vi "Configure RF Output.vi"(4 "Enable Reverse Power Protection (T:Enable)":bool=TRUE, 6 "Enable Blanking (T:Enable)":bool=TRUE, 7 "Enable Modulation (T:Enable)":bool=TRUE, 8 "error in (no error)":errorcluster, 9 "Auto Blanking (T:Enable)":bool=TRUE, 10 "Enable RF Output (F:Disable)":bool, 11 "VISA resource name":refnum<visa-resource-name>) -> (0 "error out":errorcluster, 3 "VISA resource name out":refnum<visa-resource-name>)   [LabVIEW 2014, in "Agilent PSG MXG Series.lvlib"]
doc: "Configures RF output, modulation state, blanking, and RPP circuit of the signal generator."
uses:
  Agilent PSG MXG Series.lvlib
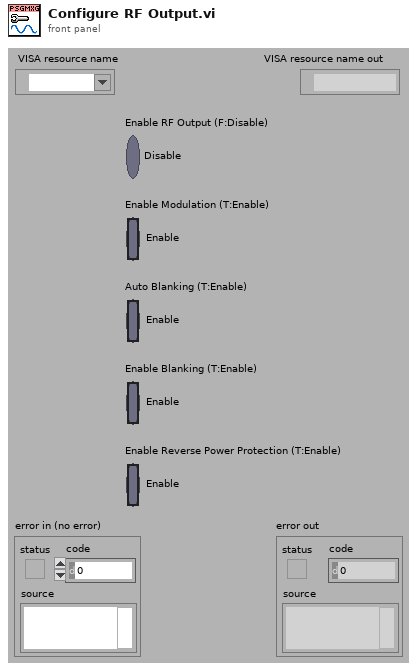
[diagram p1: front panel]
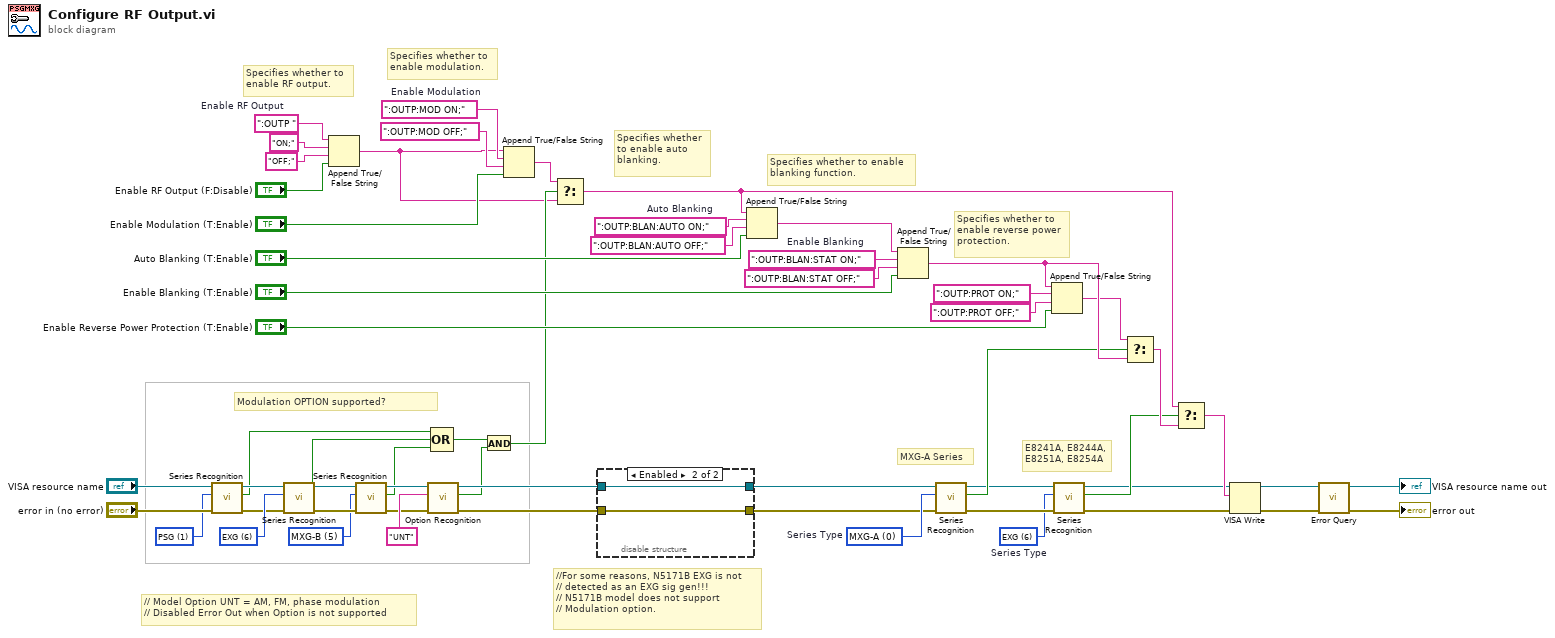
[diagram p0: block diagram]
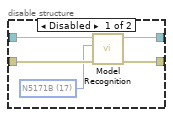
[diagram p2: hidden frame]
diagram:
  w2 = u16 1 items=["MXG-A", "PSG", "PSG-A", "PSG-C", "PSG-D", "MXG-B", "EXG"] ("Series Type (0: MXG)")
  w12 = u16 5 items=["MXG-A", "PSG", "PSG-A", "PSG-C", "PSG-D", "MXG-B", "EXG"] ("Series Type (0: MXG)")
  w23 = u16 6 items=["MXG-A", "PSG", "PSG-A", "PSG-C", "PSG-D", "MXG-B", "EXG"] ("Series Type")
  w24 = u16 6 items=["MXG-A", "PSG", "PSG-A", "PSG-C", "PSG-D", "MXG-B", "EXG"]  # Series Type
  w25 = u16 0 items=["MXG-A", "PSG", "PSG-A", "PSG-C", "PSG-D", "MXG-B", "EXG"]  # Series Type
  w36 = ":OUTP:BLAN:STAT ON;"  # Enable Blanking
  w51 = ":OUTP:BLAN:AUTO ON;"  # Auto Blanking
  w54 = ":OUTP:MOD ON;"  # Enable Modulation
  w58 = ":OUTP "  # Enable RF Output
  # "Modulation OPTION supported?"
  # "//For some reasons, N5171B EXG is not\n// detected as an EXG sig gen!!!\n// N5171B model does not support\n// Modulation option."
  # "// Model Option UNT = AM, FM, phase modulation\n// Disabled Error Out when Option is not supported"
  # "MXG-A Series"
  # "Specifies whether to\nenable reverse power\nprotection."
  # "Specifies whether to enable\nblanking function."
  # "Specifies whether\nto enable auto\nblanking."
  # "Specifies whether to\nenable modulation."
  # "Specifies whether to\nenable RF output."
  # "E8241A, E8244A,\nE8251A, E8254A"
  n1 = call "Series Recognition.vi"("error in (no error)"="error in (no error)", "Series Type (0: MXG)"=w2, "VISA resource name"="VISA resource name") -> ("error out"=w4:errorcluster, "Is Series Correct"=w1:bool, "VISA resource name out"=w3:refnum<visa-resource-name>)  [unwired: 1 in, 5 out]
  n2 = call "Series Recognition.vi"("error in (no error)"=w4, "Series Type (0: MXG)"=w23, "VISA resource name"=w3) -> ("error out"=w16:errorcluster, "Is Series Correct"=w9:bool, "VISA resource name out"=w15:refnum<visa-resource-name>)  [unwired: 1 in, 5 out]
  n3 = Append True/False String(1:"Enable RF Output (F:Disable)", 2:"OFF;" ("false string"), 3:"ON;" ("true string"), 4:w58) -> (0:w7:string)
  n4 = call "Series Recognition.vi"("error in (no error)"=w16, "Series Type (0: MXG)"=w12, "VISA resource name"=w15) -> ("error out"=w13:errorcluster, "Is Series Correct"=w10:bool, "VISA resource name out"=w14:refnum<visa-resource-name>)  [unwired: 1 in, 5 out]
  n5 = call "Option Recognition.vi"("error in (no error)"=w13, "Option (\"\")"="UNT" ("Option (\"\")"), "VISA resource name"=w14) -> ("error out"=w19:errorcluster, "Is Option Installed"=w17:bool, "VISA resource name out"=w20:refnum<visa-resource-name>)  [unwired: 6 out]
  n6 = Compound Arithmetic op=OR(w1, w9, w10) -> (w11:bool)
  n7 = And(x=w11, y=w17) -> (x .and. y?=w18:bool)
  n8 = Append True/False String(1:"Enable Modulation (T:Enable)", 2:":OUTP:MOD OFF;" ("true string"), 3:w54, 4:w7) -> (0:w8:string)
  n9 = Select(t=w8, s=w18, f=w7) -> (s? t:f=w27:string)
  n10 = disable-structure shown="Enabled" {
    disable-tunnel: [w63 w65] -> w22
    disable-tunnel: [w62 w64] -> w21
    disable-tunnel: w20 -> [w61 w64]
    disable-tunnel: w19 -> [w60 w65]
    frame Disabled {
      w59 = u16 17 items=["N5181A"=0, "N5182A"=1, "N5183A"=2, "N5161A"=3, "N5162A"=4, "E8241A"=5, "E8244A"=6, "E8251A"=7, "E8254A"=8, "E8247C"=10, "E8257C"=11, "E8267C"=12, "E8257D"=15, "E8267D"=16, "N5171B"=17, "N5172B"=18, "N5181B"=19, "N5182B"=20] ("Model Type (0: N5181A)")
      n11 = call "Model Recognition.vi"("error in (no error)"=w60, "Model Type (0: N5181A)"=w59, "VISA resource name"=w61) -> ("error out"=w63:errorcluster, "VISA resource name out"=w62:refnum<visa-resource-name>)  [unwired: 7 out]
    }
    frame Enabled {
    }
  }
  n12 = Append True/False String(1:"Auto Blanking (T:Enable)", 2:":OUTP:BLAN:AUTO OFF;" ("true string"), 3:w51, 4:w27) -> (0:w48:string)
  n13 = Append True/False String(1:"Enable Blanking (T:Enable)", 2:":OUTP:BLAN:STAT OFF;" ("true string"), 3:w36, 4:w48) -> (0:w40:string)
  n14 = call "Series Recognition.vi"("error in (no error)"=w22, "Series Type (0: MXG)"=w25, "VISA resource name"=w21) -> ("error out"=w33:errorcluster, "Is Series Correct"=w35:bool, "VISA resource name out"=w34:refnum<visa-resource-name>)  [unwired: 1 in, 5 out]
  n15 = Append True/False String(1:"Enable Reverse Power Protection (T:Enable)", 2:":OUTP:PROT OFF;" ("true string"), 3:":OUTP:PROT ON;" ("Enable Reverse Power Protection"), 4:w40) -> (0:w39:string)
  n16 = call "Series Recognition.vi"("error in (no error)"=w33, "Series Type (0: MXG)"=w24, "VISA resource name"=w34) -> ("error out"=w30:errorcluster, "Is Series Correct"=w32:bool, "VISA resource name out"=w31:refnum<visa-resource-name>)  [unwired: 1 in, 5 out]
  n17 = Select(t=w39, s=w35, f=w40) -> (s? t:f=w38:string)
  n18 = Select(t=w27, s=w32, f=w38) -> (s? t:f=w37:string)
  n19 = VISA Write(VISA resource name=w31, write buffer=w37, error in (no error)=w30) -> (VISA resource name out=w42:refnum<visa-resource-name>, error out=w41:errorcluster)  [unwired: 1 out]
  n20 = call "Error Query.vi"("error in (no error)"=w41, "VISA resource name"=w42) -> ("error out"=→"error out":errorcluster, "VISA resource name out"=→"VISA resource name out":refnum<visa-resource-name>)  [unwired: 8 out]
